vi "printout panel.vi"(5 "Test results (spec.)":string, 7 "Print add. info":T1, 8 "error in (no error)":errorcluster, 9 "print data":T2(array[cluster]), 10 "selected printer":string, 11 "XY Graph (main VI)":refnum<vi>) -> (0 "error out":errorcluster)   [LabVIEW 2014]
uses:
  <vilib>/printing/EasyPrintingControls.llb/layout_options.ctl
  <vilib>/printing/EasyPrintingControls.llb/orientation.ctl
  <vilib>/printing/EasyPrintingControls.llb/panel_scaling_for_page.ctl
  <vilib>/printing/EasyPrintingControls.llb/margins.ctl
  <vilib>/printing/EasyPrintingControls.llb/margin_values.ctl
  <vilib>/printing/EasyPrintingControls.llb/measurement_system.ctl
  <vilib>/printing/EasyPrintingControls.llb/printer_options.ctl
  <vilib>/printing/EasyPrintingControls.llb/printing_method.ctl
  <vilib>/printing/EasyPrintingControls.llb/color_or_monochrome.ctl
  <vilib>/printing/EasyPrintingControls.llb/page_header_options.ctl
  <vilib>/printing/EasyPrintingControls.llb/page_headers.ctl
  <vilib>/printing/EasyPrintingControls.llb/page_header_content_options.ctl
  <vilib>/printing/EasyPrintingControls.llb/contents.ctl
  <vilib>/printing/EasyPrinting.llb/Easy Print VI Panel or Documentation (path).vi
  <vilib>/Utility/NIReport.llb/NI_ReportGenerationCore.lvlib
panel:
  out "Test results (spec.)":string
  out "Batch":string
  out "Run No":string
  out "Date":string
  out "Tube Type":string
  in  "layout options":T3={"orientation (unchanged)"=0, "panel scaling for page (unchanged)"=0, "margins"={"override VI margins (false)"=FALSE, "margins (1.00)"={"top"=1.0, "left"=1.0, "right"=1.0, "bottom"=1.0}, "measurement system (default)"=0}, "printer options"={"destination printer name (current)"="", "printing method (unchanged)"=0, "color or monochrome (unchanged)"=0}, "page header options"={"page headers (unchanged)"=0, "page header content options"={"Include VI Name"=TRUE, "Include VI Path"=TRUE, "Include Last Modification Date"=TRUE, "Include Date Printed"=TRUE, "Include Page Number"=TRUE, "Include VI Icon"=TRUE}}} {"page header options"."page headers (unchanged)" items=["Unchanged", "Include page headers", "Do not include page headers"]; "printer options"."color or monochrome (unchanged)" items=["Unchanged", "Color/grayscale", "Monochrome"]; "printer options"."printing method (unchanged)" items=["Unchanged", "Standard", "PostScript", "Bitmap"]; "panel scaling for page (unchanged)" items=["Unchanged", "No Scaling", "Scale front panel to fit"]; "orientation (unchanged)" items=["Unchanged", "portrait", "landscape"]; "margins"."measurement system (default)" items=["Default", "US", "Metric"]; "margins"."margins (1.00)"."right" format="%.2f"; "margins"."margins (1.00)"."bottom" format="%.2f"; "margins"."margins (1.00)"."top" format="%.2f"; "margins"."margins (1.00)"."left" format="%.2f"}
  out "XY Graph (print)":T15(graph)
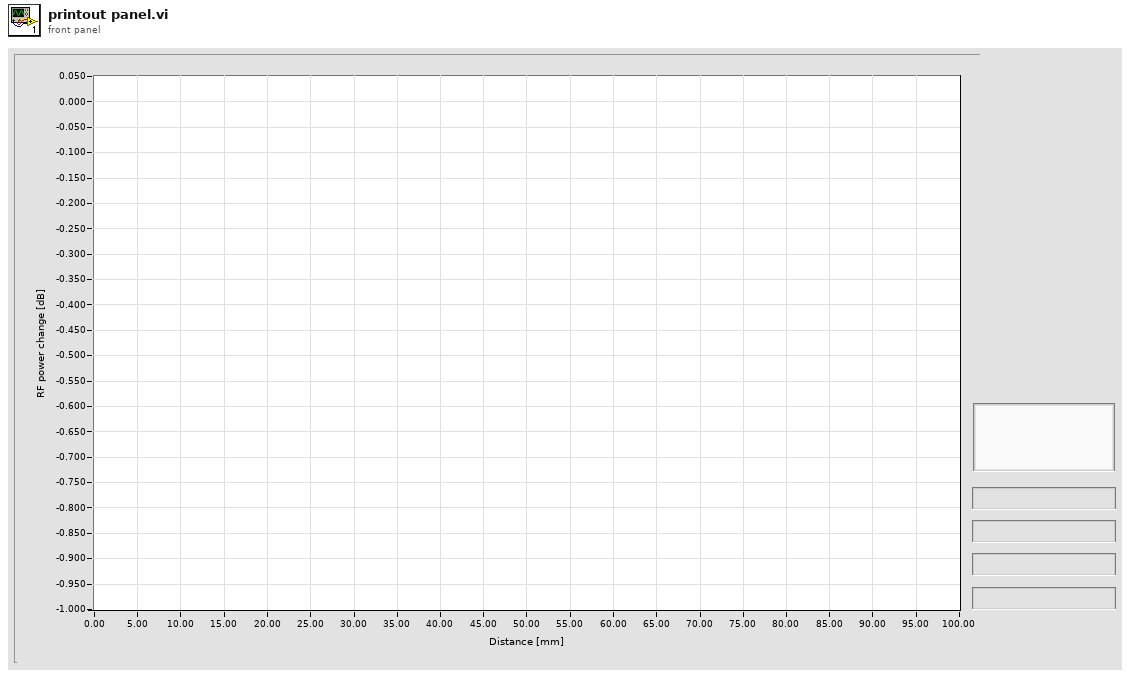
[diagram p1: front panel]
types:
  T1 = cluster{"Tube Type":string, "Date":string, "Run No":string, "Batch":string}
  T2 = cluster{"plot 3 data":dbl[], "plot 3 data":dbl[]}[]
  T3 = typedef "NI_ReportGenerationCore.lvlib/layout_options.ctl" = cluster{"orientation (unchanged)":T4, "panel scaling for page (unchanged)":T5, "margins":T6, "printer options":T9, "page header options":T12}
  T4 = typedef "NI_ReportGenerationCore.lvlib/orientation.ctl" = u16
  T5 = typedef "NI_ReportGenerationCore.lvlib/panel_scaling_for_page.ctl" = u16
  T6 = typedef "NI_ReportGenerationCore.lvlib/margins.ctl" = cluster{"override VI margins (false)":bool, "margins (1.00)":T7, "measurement system (default)":T8}
  T7 = typedef "NI_ReportGenerationCore.lvlib/margin_values.ctl" = cluster{"top":dbl, "left":dbl, "right":dbl, "bottom":dbl}
  T8 = typedef "NI_ReportGenerationCore.lvlib/measurement_system.ctl" = u16
  T9 = typedef "NI_ReportGenerationCore.lvlib/printer_options.ctl" = cluster{"destination printer name (current)":string, "printing method (unchanged)":T10, "color or monochrome (unchanged)":T11}
  T10 = typedef "NI_ReportGenerationCore.lvlib/printing_method.ctl" = u16
  T11 = typedef "NI_ReportGenerationCore.lvlib/color_or_monochrome.ctl" = u16
  T12 = typedef "NI_ReportGenerationCore.lvlib/page_header_options.ctl" = cluster{"page headers (unchanged)":T13, "page header content options":T14}
  T13 = typedef "NI_ReportGenerationCore.lvlib/page_headers.ctl" = u16
  T14 = typedef "NI_ReportGenerationCore.lvlib/page_header_content_options.ctl" = cluster{"Include VI Name":bool, "Include VI Path":bool, "Include Last Modification Date":bool, "Include Date Printed":bool, "Include Page Number":bool, "Include VI Icon":bool}
  T15 = cluster{"plot 1 data":dbl[], "plot 1 data":dbl[]}[]
  T16 = typedef "NI_ReportGenerationCore.lvlib/contents.ctl" = u16
  T17 = typedef "LVCursorListTypeDef.ctl" = cluster{"Name":string, "Color":u32, "Style":u8, "Point Style":u8, "Name Visible":bool, "Allow Drag":bool, "Cursor Mode":u32, "Plot":i32, "Index":i32, "Position":cluster{"X":dbl, "Y":dbl}, "X Scale":u32, "Y Scale":u32, "Watch Plots":i32[], "Watch All Plots":bool, "Plot Area":i32, "Label Offset":cluster{"X":dbl, "Y":dbl}}[]
  T18 = typedef "LVAnnotationListTypeDef.ctl" = cluster{"Name":string, "Color":u32, "Style":u8, "Point Style":u8, "Name Visible":bool, "Allow Drag":bool, "Annotation Mode":u32, "Plot":i32, "Index":i32, "Position":cluster{"X":dbl, "Y":dbl}, "X Scale":u32, "Y Scale":u32, "Show Arrow":bool, "Lock Name":bool, "Plot Area":i32, "Label Offset":cluster{"X":dbl, "Y":dbl}}[]
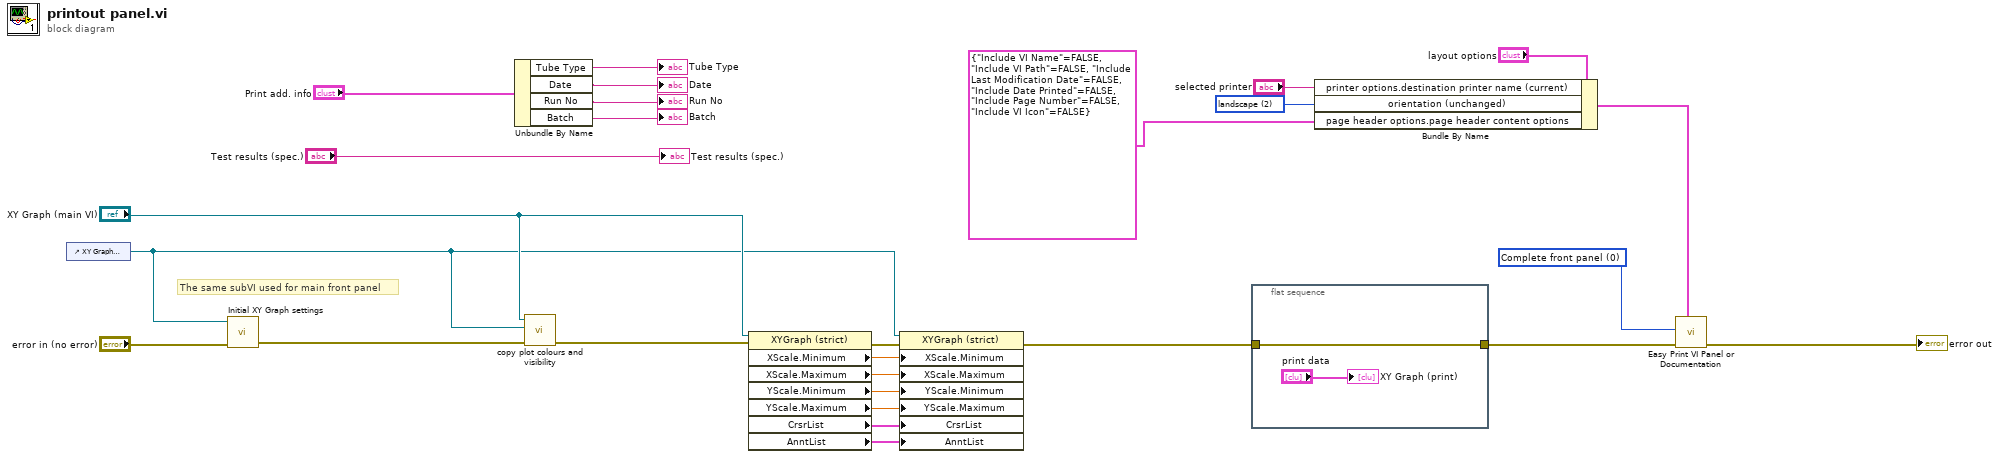
[diagram p0: block diagram]
diagram:
  w14 = T16 0 items=["Complete front panel", "Visible portion of front panel", "Icon, description, panel and diagram", "Documentation: Using the panel", "Documentation: Using as a subVI", "Documentation: Complete", "Documentation: Custom"] ("contents (complete front panel)")
  w15 = T4 2 items=["Unchanged", "portrait", "landscape"] ("orientation (unchanged)")
  # "The same subVI used for main front panel"
  n1 = control-ref of="XY Graph (print)"() -> (w2:refnum<vi>)
  n2 = call "Initial XY Graph settings.vi"("error in (no error)"="error in (no error)", "XYGraph in"=w2) -> ("error out"=w5:errorcluster)  [unwired: 9 in]
  n3 = Unbundle By Name("Print add. info") -> ("Tube Type"=→"Tube Type":string, "Date"=→"Date":string, "Run No"=→"Run No":string, "Batch"=→"Batch":string)
  n4 = call "copy plot colours and visibility.vi"("error in"=w5, "XY Graph (print)"=w2, "XY Graph (main VI)"="XY Graph (main VI)") -> ("error out"=w4:errorcluster)  [unwired: 8 in]
  n5 = property class="XYGraph (strict)"(reference="XY Graph (main VI)", error in=w4) -> (error out=w23:errorcluster, "XScale.Minimum"=w19:dbl, "XScale.Maximum"=w20:dbl, "YScale.Minimum"=w18:dbl, "YScale.Maximum"=w17:dbl, "CrsrList"=w16:T17, "AnntList"=w6:T18)  [unwired: 1 out]
  n6 = property on="Property Node" class="XYGraph (strict)"(reference=w2, error in=w23, "XScale.Minimum"=w19, "XScale.Maximum"=w20, "YScale.Minimum"=w18, "YScale.Maximum"=w17, "CrsrList"=w16, "AnntList"=w6) -> (error out=w22:errorcluster)  [unwired: 1 out]
  n7 = flat-sequence {
    tunnel: w22 -> [w29]
    tunnel: [w29] -> w21
    frame #0 {
      "XY Graph (print)" <- "print data"
    }
  }
  n8 = Bundle By Name(cluster="layout options", "printer options.destination printer name (current)"="selected printer", "orientation (unchanged)"=w15, "page header options.page header content options"=T14 {"Include VI Name"=FALSE, "Include VI Path"=FALSE, "Include Last Modification Date"=FALSE, "Include Date Printed"=FALSE, "Include Page Number"=FALSE, "Include VI Icon"=FALSE}) -> (w26:T3)
  n9 = call-poly <vilib>:"Easy Print VI Panel or Documentation.vi"("layout options"=w26, "error in (no error)"=w21, "contents (complete front panel)"=w14) -> ("error out"=→"error out":errorcluster)  [unwired: 7 in, 1 out]
  "Test results (spec.)" <- "Test results (spec.)"
